vi "Read ForceFollowCycle.vi"(8 "error in (no error)":errorcluster, 11 "AI_Snake in":refnum<class "AI_Snake.lvclass">) -> (0 "error out":errorcluster, 2 "ForceFollowCycle":bool, 3 "AI_Snake out":refnum<class "AI_Snake.lvclass">)   [LabVIEW 2019, in "RT_Game.lvlib" / "AI_Snake.lvclass"]
uses:
  AI_Snake.lvclass
  AI_Snake.lvclass/AI_Snake.ctl
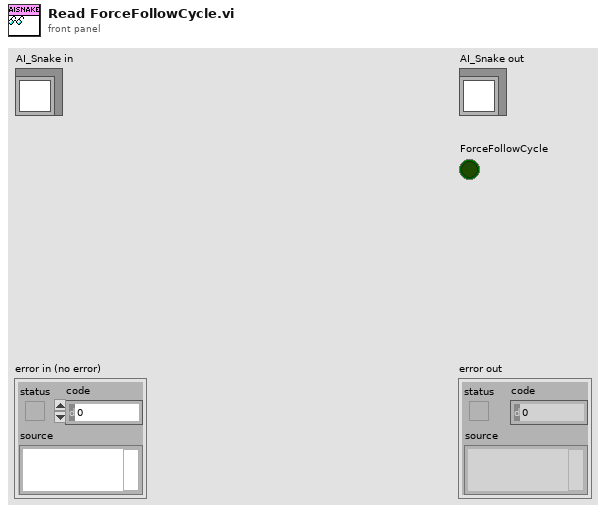
[diagram p1: front panel]
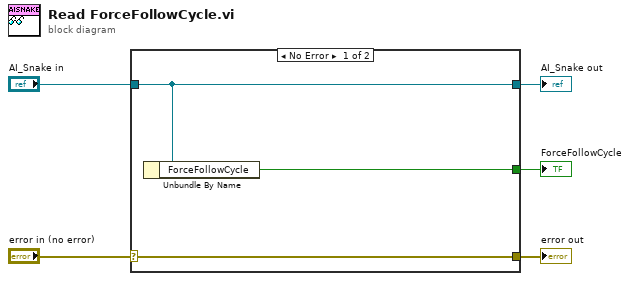
[diagram p0: block diagram]
diagram:
  n1 = case shown="No Error" "error in (no error)" {
    selector: "error in (no error)" -> [w8 w9]
    tunnel: [w8 w9] -> w4
    tunnel: [w7 w10] -> w2
    tunnel: "AI_Snake in" -> [w7 w10]
    tunnel: [w6 _] -> w1
    frame No Error {
      n2 = Unbundle By Name(w7) -> ("ForceFollowCycle"=w6:bool)
    }
    frame Error {
    }
  }
  "error out" <- w4
  "AI_Snake out" <- w2
  "ForceFollowCycle" <- w1
